vi "GOOP_XControl_Item_OnCommand.vi"(10 "Command Tag":string, 11 "Object":u64) -> ()   [LabVIEW 2020]
uses:
  <resource>/Framework/Providers/Open_GDS/SubVIs/GOOP_UMLEditor_CallMainAction.ctl
  <resource>/Framework/Providers/Open_GDS/ClassProviders/Provider_BaseClassInterface/ClassWriter_class/ClassWriter.lvclass
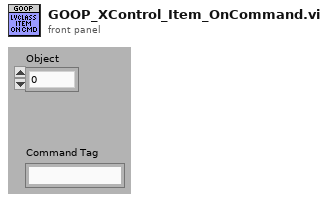
[diagram p1: front panel]
types:
  T1 = typedef "GOOP_UMLEditor_CallMainAction.ctl" = enum16{"OpenUmlEditor", "ReverseEngineering:WholeProject", "ReverseEngineering:OneClass", "ReverseEngineering:OneVI", "ShowInStateDiagram:OneVI", "OpenUMLFile"}
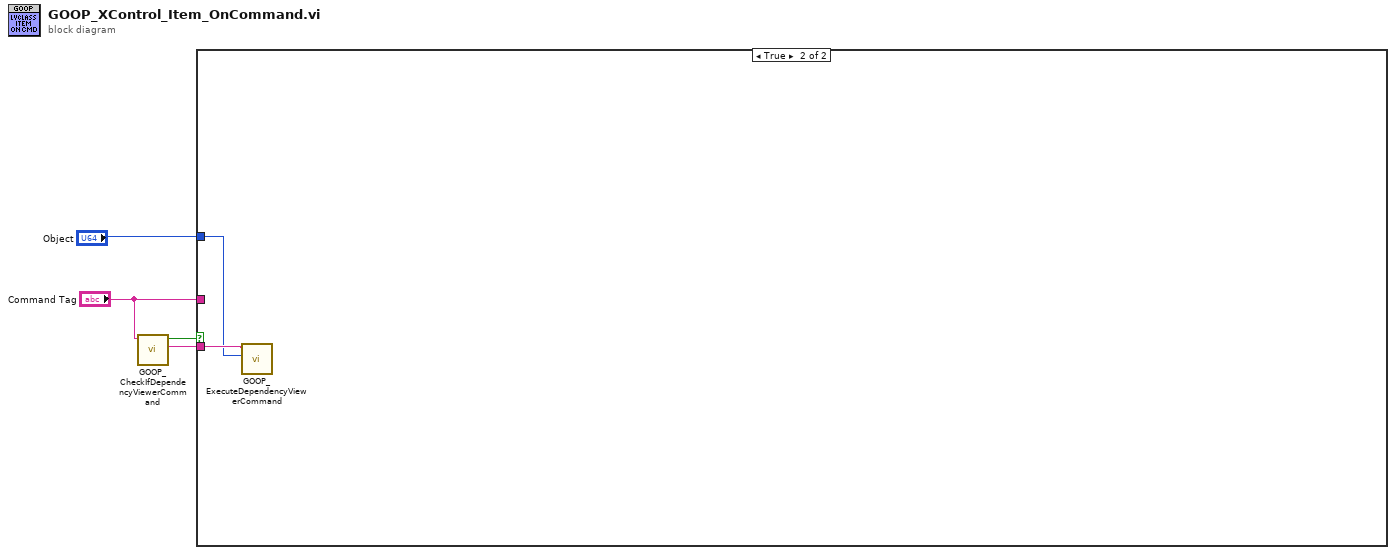
[diagram p0: block diagram]
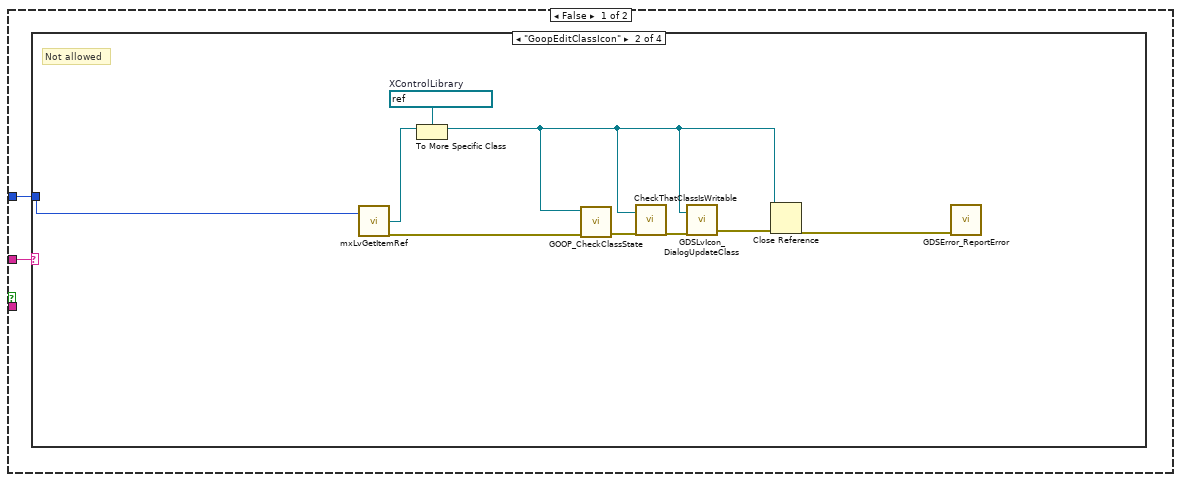
[diagram p2: hidden frame]
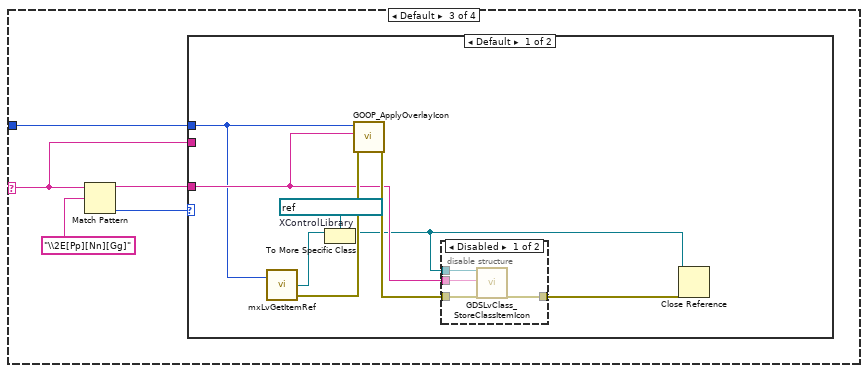
[diagram p4: hidden frame]
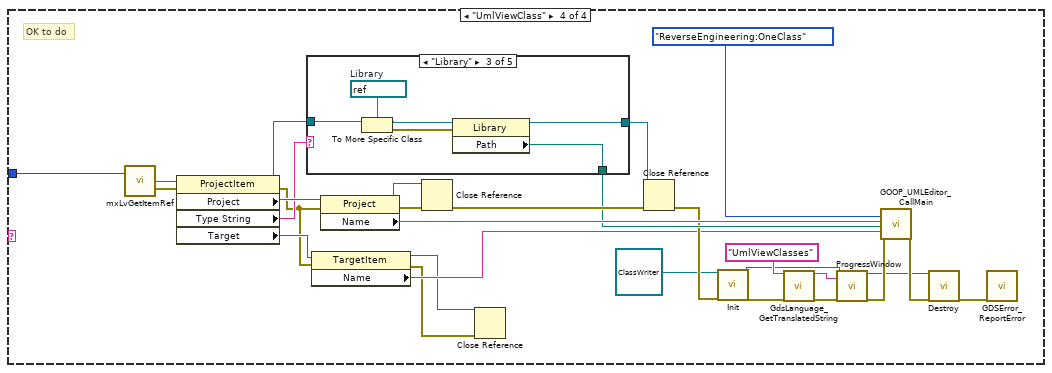
[diagram p7: hidden frame]
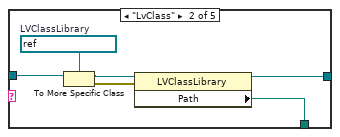
[diagram p9: hidden frame]
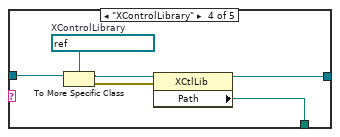
[diagram p10: hidden frame]
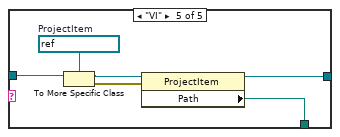
[diagram p11: hidden frame]
diagram:
  n1 = call <resource>:"GOOP_CheckIfDependencyViewerCommand.vi"("Command Tag"="Command Tag") -> ("Sub Command"=w1:string, "Is It a Dependency Viewer Command"=w2:bool)  [unwired: 9 in]
  n2 = case shown="True" w2 {
    tunnel: "Object" -> [w6 w88]
    tunnel: "Command Tag" -> [w5 _]
    tunnel: w1 -> [_ w89]
    frame False {
      n3 = case shown="\"GoopEditClassIcon\"" w5 {
        selector: w5 -> [_ _ w18 _]
        tunnel: w6 -> [_ w14 w19 w39]
        frame "False" {
        }
        frame "GoopEditClassIcon" {
          w15 = refnum<vi> refnum  # XControlLibrary
          # "Not allowed"
          n4 = call <resource>:"mxLvGetItemRef.vi"("Item"=w14) -> ("Item Refnum"=w13:refnum<vi>, "error out"=w8:errorcluster)  [unwired: 1 in, 1 out]
          n5 = To More Specific Class(target class=w15, reference=w13) -> (specific class reference=w7:refnum<vi>)  [unwired: 1 in, 1 out]
          n6 = call <resource>:"GOOP_CheckClassState.vi"("error in"=w8, "Library Refnum"=w7) -> ("error out"=w9:errorcluster)  [unwired: 9 in]
          n7 = call <resource>:"CheckThatClassIsWritable.vi"("Library Refnum"=w7, "error in (no error)"=w9) -> ("error out"=w10:errorcluster)  [unwired: 16 in, 1 out]
          n8 = call <resource>:"GDSLvIcon_DialogUpdateClass.vi"("ClassPath(FilePath/ProjectTreePath/LvCLassRef)"=w7, "error in (no error)"=w10) -> ("error out"=w12:errorcluster)  [unwired: 14 in, 3 out]
          n9 = Close Reference(reference=w7, error in (no error)=w12) -> (error out=w11:errorcluster)
          n10 = call <resource>:"GDSError_ReportError.vi"("error in (no error)"=w11) -> ()  [unwired: 18 in, 1 out]
        }
        frame Default {
          n11 = Match Pattern(string=w18, regular expression="\\2E[Pp][Nn][Gg]") -> (before substring=w16:string, offset past match=w17:i32)  [unwired: 1 in, 2 out]
          n12 = case shown="Default" w17 {
            tunnel: w19 -> [w22 _]
            tunnel: w18 -> [_ _]
            tunnel: w16 -> [w23 _]
            frame Default {
              w28 = refnum<vi> refnum  # XControlLibrary
              n13 = call <resource>:"mxLvGetItemRef.vi"("Item"=w22) -> ("Item Refnum"=w27:refnum<vi>, "error out"=w26:errorcluster)  [unwired: 1 in, 1 out]
              n14 = To More Specific Class(target class=w28, reference=w27) -> (specific class reference=w21:refnum<vi>)  [unwired: 1 in, 1 out]
              n15 = call <resource>:"GOOP_ApplyOverlayIcon.vi"("error in (no error)"=w26, "IconName(NoPngExtension)"=w23, "Object"=w22) -> ("error out"=w25:errorcluster)  [unwired: 8 in]
              n16 = disable-structure shown="Disabled" {
                disable-tunnel: w25 -> [w32 w33]
                disable-tunnel: [w31 w33] -> w24
                disable-tunnel: w23 -> [w30 _]
                disable-tunnel: w21 -> [w29 _]
                frame Disabled {
                  n17 = call <resource>:"GDSLvClass_StoreClassItemIcon.vi"("Library Refnum"=w29, "ClassItemIconName"=w30, "error in (no error)"=w32) -> ("error out"=w31:errorcluster)  [unwired: 15 in, 1 out]
                }
                frame Enabled {
                }
              }
              n18 = Close Reference(reference=w21, error in (no error)=w24) -> ()  [unwired: 1 out]
            }
            frame -1 {
            }
          }
        }
        frame "UmlViewClass" {
          # "OK to do"
          n19 = call <resource>:"mxLvGetItemRef.vi"("Item"=w39) -> ("Item Refnum"=w61:refnum<vi>, "error out"=w51:errorcluster)  [unwired: 1 in, 1 out]
          n20 = property class="ProjectItem"(reference=w61, error in=w51) -> (reference out=w55:refnum<vi>, error out=w34:errorcluster, "Project"=w60:refnum<vi>, "Type String"=w53:string, "Target"=w38:refnum<vi>)
          n21 = case shown="\"Library\"" w53 {
            tunnel: w55 -> [w63 w69 w75 w81 w87]
            tunnel: [w63 w65 w71 w77 w83] -> w54
            tunnel: [_ w64 w70 w76 w82] -> w52
            frame Default {
            }
            frame "LvClass" {
              w68 = refnum<vi> refnum  # LVClassLibrary
              n22 = To More Specific Class(target class=w68, reference=w69) -> (specific class reference=w67:refnum<vi>, error out=w66:errorcluster)  [unwired: 1 in]
              n23 = property class="LVClassLibrary"(reference=w67, error in=w66) -> (reference out=w65:refnum<vi>, "Path"=w64:path)  [unwired: 1 out]
            }
            frame "Library" {
              w74 = refnum<vi> refnum  # Library
              n24 = To More Specific Class(target class=w74, reference=w75) -> (specific class reference=w73:refnum<vi>, error out=w72:errorcluster)  [unwired: 1 in]
              n25 = property class="Library"(reference=w73, error in=w72) -> (reference out=w71:refnum<vi>, "Path"=w70:path)  [unwired: 1 out]
            }
            frame "XControlLibrary" {
              w80 = refnum<vi> refnum  # XControlLibrary
              n26 = To More Specific Class(target class=w80, reference=w81) -> (specific class reference=w79:refnum<vi>, error out=w78:errorcluster)  [unwired: 1 in]
              n27 = property class="XCtlLib"(reference=w79, error in=w78) -> (reference out=w77:refnum<vi>, "Path"=w76:path)  [unwired: 1 out]
            }
            frame "VI" {
              w86 = refnum<vi> refnum  # ProjectItem
              n28 = To More Specific Class(target class=w86, reference=w87) -> (specific class reference=w85:refnum<vi>, error out=w84:errorcluster)  [unwired: 1 in]
              n29 = property class="ProjectItem"(reference=w85, error in=w84) -> (reference out=w83:refnum<vi>, "Path"=w82:path)  [unwired: 1 out]
            }
          }
          n30 = property class="TargetItem"(reference=w38, error in=w34) -> (reference out=w36:refnum<vi>, error out=w35:errorcluster, "Name"=w37:string)
          n31 = property class="Project"(reference=w60, error in=w34) -> (reference out=w57:refnum<vi>, error out=w58:errorcluster, "Name"=w59:string)
          n32 = Close Reference(reference=w57, error in (no error)=w58) -> (error out=w56:errorcluster)
          n33 = Close Reference(reference=w36, error in (no error)=w35) -> ()  [unwired: 1 out]
          n34 = Close Reference(reference=w54, error in (no error)=w56) -> (error out=w47:errorcluster)
          n35 = call-dynamic "Init.vi"("ClassWriter in"=refnum<class "ClassWriter.lvclass"> refnum, "error in (no error)"=w47) -> ("ClassWriter out"=w42:refnum<class "ClassWriter.lvclass">, "error out"=w46:errorcluster)  [unwired: 16 in]
          n36 = call <resource>:"GdsLanguage_GetTranslatedString.vi"("StringID(s)"="UmlViewClasses" ("Message(Exit)"), "error in (no error)"=w46) -> ("FirstStringOut"=w50:string, "error out"=w49:errorcluster)  [unwired: 14 in, 2 out]
          n37 = call-dynamic "ProgressWindow.vi"("ClassWriter in"=w42, "Message(Exit)"=w50, "error in (no error)"=w49) -> ("ClassWriter out"=w43:refnum<class "ClassWriter.lvclass">, "error out"=w45:errorcluster)  [unwired: 15 in]
          n38 = call <resource>:"GOOP_UMLEditor_CallMain.vi"("Enum"=GOOP_UMLEditor_CallMainAction."ReverseEngineering:OneClass", "Project"=w59, "Class/VI-Path"=w52, "Target"=w37, "error in (no error)"=w45) -> ("error out"=w44:errorcluster)  [unwired: 14 in]
          n39 = call-dynamic "Destroy.vi"("ClassWriter.lvclass"=w43, "error in (no error)"=w44) -> ("error out"=w41:errorcluster)  [unwired: 17 in]
          n40 = call <resource>:"GDSError_ReportError.vi"("error in (no error)"=w41) -> ()  [unwired: 18 in, 1 out]
        }
      }
    }
    frame True {
      n41 = call <resource>:"GOOP_ExecuteDependencyViewerCommand.vi"("Object"=w88, "Sub Command"=w89) -> ()  [unwired: 10 in]
    }
  }
